vi "triggertest2.vi"(11 "trigger in":bool) -> (3 "trigger out":bool)   [LabVIEW 2020]
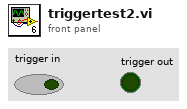
[diagram p1: front panel]
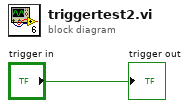
[diagram p0: block diagram]
diagram:
  "trigger out" <- "trigger in"
